vi "Q-View.vi"(7 "Queue Type":T3, 8 "error in":errorcluster, 10 "Return Elements? (F)":bool, 11 "Q Name":string) -> (0 "error out":errorcluster, 1 "Analog data":T5(array[cluster]), 2 "Q-Info":T4, 3 "Digital Data":T1(array[cluster]), 5 "Variant Data":T2(array[cluster]))   [LabVIEW 2016]
uses:
  PSDAQEG_Task Queue Type.ctl
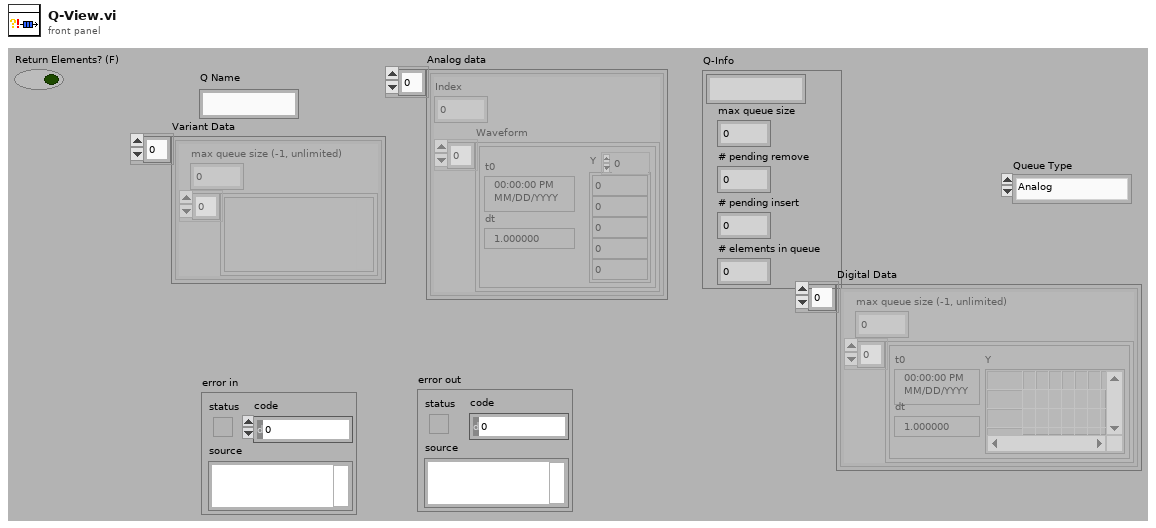
[diagram p1: front panel]
types:
  T1 = cluster{"max queue size (-1, unlimited)":i32, digitalwaveform[]}[]
  T2 = cluster{"max queue size (-1, unlimited)":i32, variant[]}[]
  T3 = typedef "PSDAQEG_Task Queue Type.ctl" = enum16{"Analog", "Digital", "Variant"}
  T4 = cluster{string, "max queue size":i32, "# pending remove":i32, "# pending insert":i32, "# elements in queue":i32}
  T5 = cluster{"Index":i32, "Waveform":waveform(dbl)[]}[]
  T6 = cluster{"max queue size (-1, unlimited)":i32, "Waveform":waveform(dbl)[]}
  T7 = cluster{"max queue size (-1, unlimited)":i32, digitalwaveform[]}
  T8 = cluster{"max queue size (-1, unlimited)":i32, variant[]}
  T9 = cluster{"max queue size (-1, unlimited)":i32, "Waveform":waveform(dbl)[]}[]
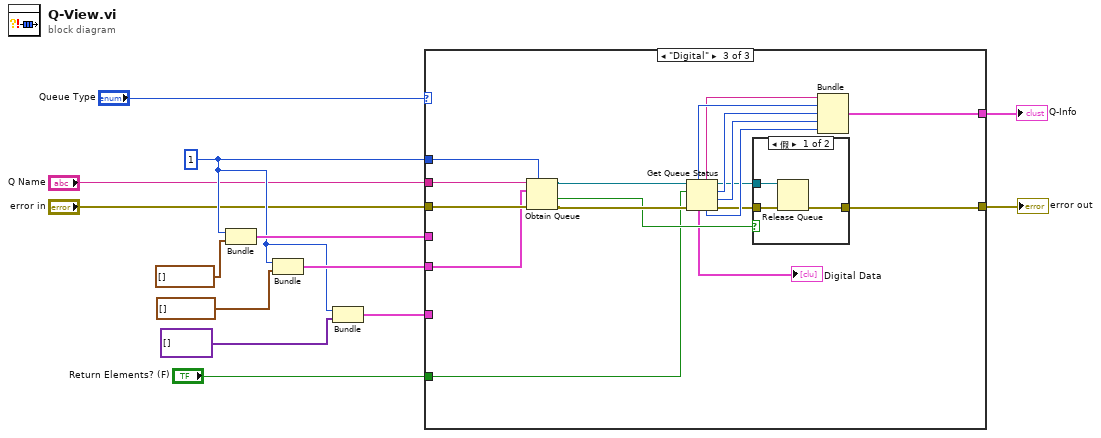
[diagram p0: block diagram]
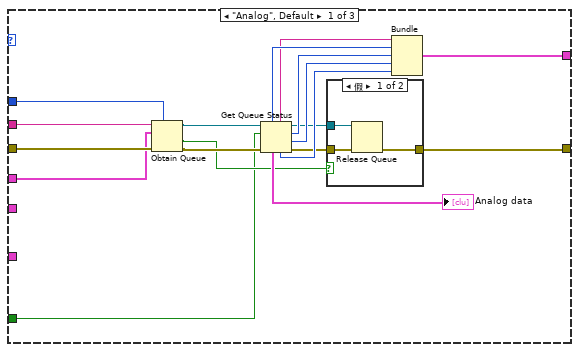
[diagram p2: hidden frame]
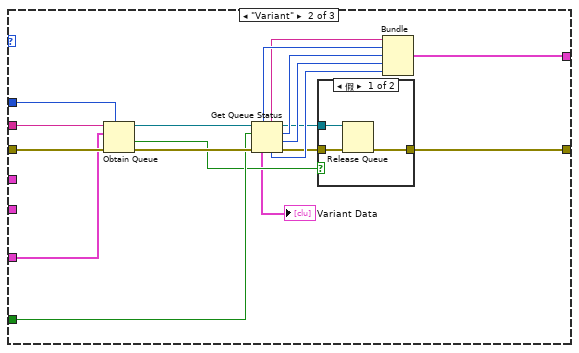
[diagram p4: hidden frame]
diagram:
  w7 = 1 ("max queue size (-1, unlimited)")
  n1 = Bundle("max queue size (-1, unlimited)"=w7, "Waveform"=waveform(dbl)[] []) -> (w9:T6)  [unwired: 1 in]
  n2 = Bundle("max queue size (-1, unlimited)"=w7, digitalwaveform[] []) -> (w10:T7)  [unwired: 1 in]
  n3 = Bundle("max queue size (-1, unlimited)"=w7, variant[] []) -> (w6:T8)  [unwired: 1 in]
  n4 = case shown="\"Digital\"" "Queue Type" {
    tunnel: "Q Name" -> [w30 w52 w75]
    tunnel: "error in" -> [w31 w53 w74]
    tunnel: w7 -> [w29 w51 w73]
    tunnel: w10 -> [_ _ w72]
    tunnel: [w17 w40 w62] -> w3
    tunnel: w9 -> [w28 _ _]
    tunnel: w6 -> [_ w50 _]
    tunnel: "Return Elements? (F)" -> [w15 w38 w59]
    tunnel: [w14 w39 w61] -> w1
    frame "Analog", Default {
      n5 = Obtain Queue(max queue size (-1, unlimited)=w29, name (unnamed)=w30, element data type=w28, error in (no error)=w31) -> (queue out=w19:refnum<queue>, created new?=w16:bool, error out=w18:errorcluster)  [unwired: 1 in]
      n6 = Get Queue Status(queue=w19, return elements? (F)=w15, error in (no error)=w18) -> (queue out=w20:refnum<queue>, queue name=w22:string, max queue size=w23:i32, # pending remove=w24:i32, # pending insert=w25:i32, error out=w21:errorcluster, # elements in queue=w26:i32, elements=→"Analog data":T9)
      n7 = case shown="假" w16 {
        tunnel: w20 -> [w34 _]
        tunnel: w21 -> [w33 w35]
        tunnel: [w32 w35] -> w17
        frame False {
          n8 = Release Queue(queue=w34, error in (no error)=w33) -> (error out=w32:errorcluster)  [unwired: 1 in, 2 out]
        }
        frame True {
        }
      }
      n9 = Bundle(w22, "max queue size"=w23, "# pending remove"=w24, "# pending insert"=w25, "# elements in queue"=w26) -> (w14:T4)  [unwired: 1 in]
    }
    frame "Variant" {
      n10 = Obtain Queue(max queue size (-1, unlimited)=w51, name (unnamed)=w52, element data type=w50, error in (no error)=w53) -> (queue out=w41:refnum<queue>, created new?=w37:bool, error out=w42:errorcluster)  [unwired: 1 in]
      n11 = Get Queue Status(queue=w41, return elements? (F)=w38, error in (no error)=w42) -> (queue out=w43:refnum<queue>, queue name=w45:string, max queue size=w46:i32, # pending remove=w47:i32, # pending insert=w48:i32, error out=w44:errorcluster, # elements in queue=w49:i32, elements=→"Variant Data":T2)
      n12 = case shown="假" w37 {
        tunnel: w43 -> [w56 _]
        tunnel: w44 -> [w55 w57]
        tunnel: [w54 w57] -> w40
        frame False {
          n13 = Release Queue(queue=w56, error in (no error)=w55) -> (error out=w54:errorcluster)  [unwired: 1 in, 2 out]
        }
        frame True {
        }
      }
      n14 = Bundle(w45, "max queue size"=w46, "# pending remove"=w47, "# pending insert"=w48, "# elements in queue"=w49) -> (w39:T4)  [unwired: 1 in]
    }
    frame "Digital" {
      n15 = Obtain Queue(max queue size (-1, unlimited)=w73, name (unnamed)=w75, element data type=w72, error in (no error)=w74) -> (queue out=w64:refnum<queue>, created new?=w60:bool, error out=w63:errorcluster)  [unwired: 1 in]
      n16 = Get Queue Status(queue=w64, return elements? (F)=w59, error in (no error)=w63) -> (queue out=w65:refnum<queue>, queue name=w67:string, max queue size=w68:i32, # pending remove=w69:i32, # pending insert=w70:i32, error out=w66:errorcluster, # elements in queue=w71:i32, elements=→"Digital Data":T1)
      n17 = case shown="假" w60 {
        tunnel: w65 -> [w78 _]
        tunnel: w66 -> [w77 w79]
        tunnel: [w76 w79] -> w62
        frame False {
          n18 = Release Queue(queue=w78, error in (no error)=w77) -> (error out=w76:errorcluster)  [unwired: 1 in, 2 out]
        }
        frame True {
        }
      }
      n19 = Bundle(w67, "max queue size"=w68, "# pending remove"=w69, "# pending insert"=w70, "# elements in queue"=w71) -> (w61:T4)  [unwired: 1 in]
    }
  }
  "error out" <- w3
  "Q-Info" <- w1
